vi "3.4.vi"() -> ()   [LabVIEW 2017]
panel:
  in  "距离顶部":dbl=930.0 min=920.0 max=945.0 step=1.0
  in  "距离左侧":dbl=292.0 min=230.0 max=320.0 step=1.0
  in  "宽度":dbl=269.0 min=30.0 max=280.0 step=1.0
  in  "高度":dbl=30.0 min=25.0 max=50.0 step=1.0
  in  "焦点（须在可用前提下）":bool
  in  "闪烁":bool
  in  "可用":bool
  in  "可视":bool=TRUE
  in  "字符串":string
  in  "长按停止":bool
  # "任务四"
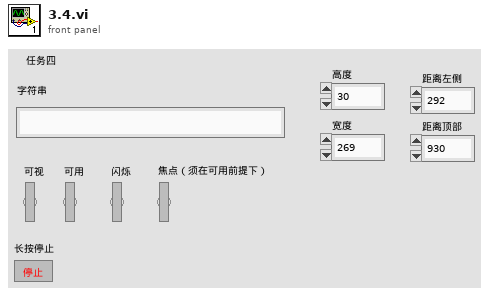
[diagram p1: front panel]
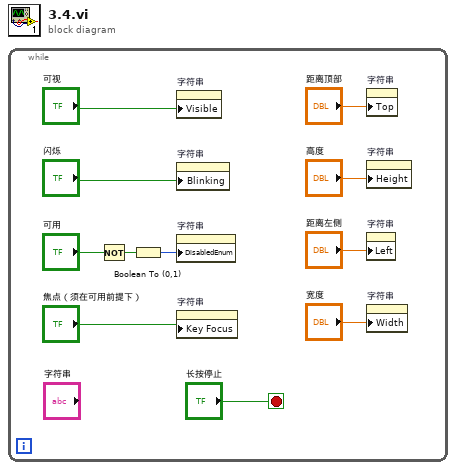
[diagram p0: block diagram]
diagram:
  n1 = while {
    stop <- "长按停止" stop-if-true
    n2 = Not(x="可用") -> (.not. x?=w8:bool)
    n3 = Boolean To (0,1)(Boolean=w8) -> (0, 1=w9:i16)
    n4 = property on="字符串" class="Str"("Visible"="可视") -> ()  [unwired: 2 in, 2 out]
    n5 = property on="字符串" class="Str"("Blinking"="闪烁") -> ()  [unwired: 2 in, 2 out]
    n6 = property on="字符串" class="Str"("DisabledEnum"=w9) -> ()  [unwired: 2 in, 2 out]
    n7 = property on="字符串" class="Str"("Key Focus"="焦点（须在可用前提下）") -> ()  [unwired: 2 in, 2 out]
    n8 = property on="字符串" class="Str"("Top"="距离顶部") -> ()  [unwired: 2 in, 2 out]
    n9 = property on="字符串" class="Str"("Height"="高度") -> ()  [unwired: 2 in, 2 out]
    n10 = property on="字符串" class="Str"("Left"="距离左侧") -> ()  [unwired: 2 in, 2 out]
    n11 = property on="字符串" class="Str"("Width"="宽度") -> ()  [unwired: 2 in, 2 out]
  }
